vi "test.vi"() -> ()   [LabVIEW 2016]
uses:
  Electrometer/Electrometer.lvclass
  ElectrometerConfiguration/ElectrometerCOMConfiguration.lvclass
panel:
  out "Measurement Function (0: Current)":i32(ring) items=["Current", "Charge", "Voltage", "Resistance"]
  out "Waveform Chart":dbl(graph)
  in  "stop":bool
  out "error out":errorcluster
  in  "VISA":refnum<visa-resource-name>
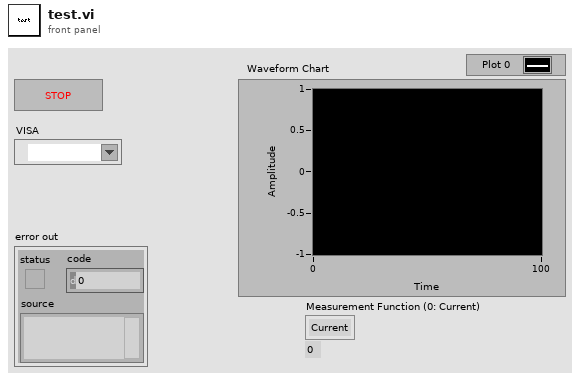
[diagram p1: front panel]
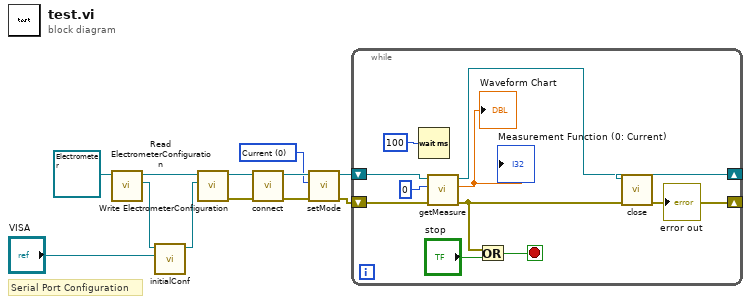
[diagram p0: block diagram]
diagram:
  w1 = 0 items=["Current", "Charge", "Voltage", "Resistance"] ("Measurement Function (0: Current)")
  # "Serial Port Configuration"
  n1 = call "Read ElectrometerConfiguration.vi"("Electrometer in"=refnum<class "Electrometer.lvclass"> refnum ("Electrometer.lvclass")) -> ("ElectrometerConfiguration"=w14:refnum<class "ElectrometerCOMConfiguration.lvclass">, "Electrometer out"=w11:refnum<class "Electrometer.lvclass">)  [unwired: 8 in, 1 out]
  n2 = call "initialConf.vi"("VISA"="VISA", "ElectrometerConfiguration In"=w14) -> ("ElectrometerConfiguration Out"=w12:refnum<class "ElectrometerCOMConfiguration.lvclass">)  [unwired: 9 in]
  n3 = call-dynamic "Write ElectrometerConfiguration.vi"("ElectrometerConfiguration"=w12, "Electrometer in"=w11) -> ("error out"=w7:errorcluster, "Electrometer out"=w6:refnum<class "Electrometer.lvclass">)  [unwired: 8 in]
  n4 = call "connect.vi"("error in (no error)"=w7, "Electrometer in"=w6) -> ("error out"=w5:errorcluster, "Electrometer out"=w3:refnum<class "Electrometer.lvclass">)  [unwired: 7 in, 1 out]
  n5 = call "setMode.vi"("error in (no error)"=w5, "Measurement Function (0: Current)"=w1, "Electrometer in"=w3) -> ("error out"=w4:errorcluster, "Electrometer out"=w2:refnum<class "Electrometer.lvclass">)  [unwired: 7 in]
  n6 = while {
    shift-right: [w21] -> w8
    shift-left: w2 -> [w24]
    shift-right: [w17] -> w10
    shift-left: w4 -> [w23]
    stop <- w19 stop-if-true
    n7 = Wait (ms)(milliseconds to wait=u32 100) -> ()  [unwired: 1 out]
    n8 = call "getMeasure.vi"("error in (no error)"=w23, "Reading Option (0: Latest)"=0, "Electrometer in"=w24) -> ("error out"=w17:errorcluster, "Measure"=→"Waveform Chart" →"Measurement Function (0: Current)":dbl, "Electrometer out"=w21:refnum<class "Electrometer.lvclass">)  [unwired: 6 in]
    n9 = Or(x=w17, y="stop") -> (x .or. y?=w19:bool)
  }
  n10 = call "close.vi"("error in (no error)"=w10, "Electrometer in"=w8) -> ("error out"=→"error out":errorcluster)  [unwired: 8 in, 1 out]
